vi "Empty.vi"(8 "error in (no error)":errorcluster, 10 "Job state":T1, 11 "Object ref in":T2) -> (0 "error out":errorcluster, 3 "Object ref out":T2)   [LabVIEW 2013, in "SLMControl.lvlib" / "SC-Main.lvclass"]
uses:
  SC-Main.lvclass
  Object-reference.ctl
  SM1000/Job-state.ctl
  SM1000/SM1000.lvclass
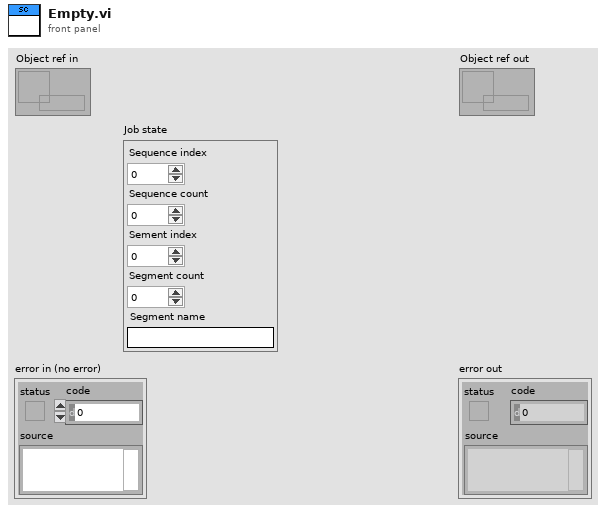
[diagram p1: front panel]
types:
  T1 = typedef "SLMControl.lvlib/SM1000.lvclass/Job-state.ctl" = cluster{"Sequence index":i32, "Sequence count":i32, "Sement index":i32, "Segment count":i32, "Segment name":string}
  T2 = typedef "SLMControl.lvlib/SC-Main.lvclass/Object-reference.ctl" = refnum<data-value>
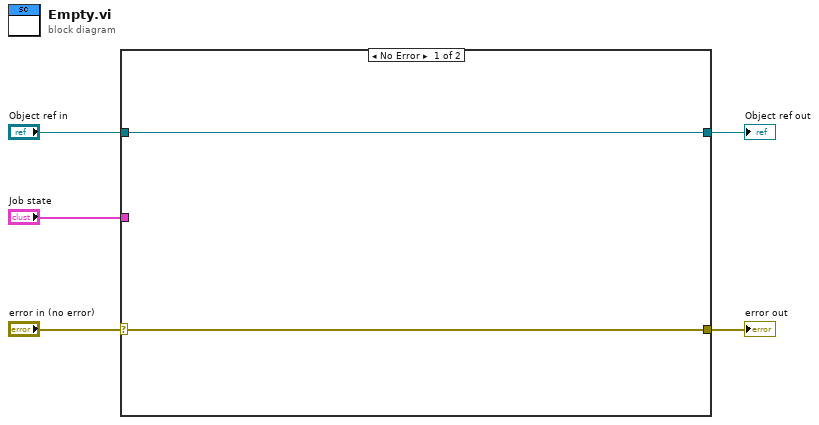
[diagram p0: block diagram]
diagram:
  n1 = case shown="No Error" "error in (no error)" {
    selector: "error in (no error)" -> [w7 w9]
    tunnel: [w7 w9] -> w4
    tunnel: [w6 w8] -> w2
    tunnel: "Object ref in" -> [w6 w8]
    tunnel: "Job state" -> [_ _]
    frame No Error {
    }
    frame Error {
    }
  }
  "error out" <- w4
  "Object ref out" <- w2
